vi "AutoMessageFGV.vi"(6 "Timeout (ms)":i32=-1, 8 "error in (no error)":errorcluster, 11 "VI Refnum In":refnum<vi>) -> (0 "error out":errorcluster, 3 "VI Refnum Out":refnum<vi>)   [LabVIEW 2019, in "MicronTemplateAPIs.lvlib" / "MicronTemplateAPIs.lvclass"]
uses:
  MicronTemplateAPIs.lvclass
  <vilib>/LabJSON/LabJSON.lvlib
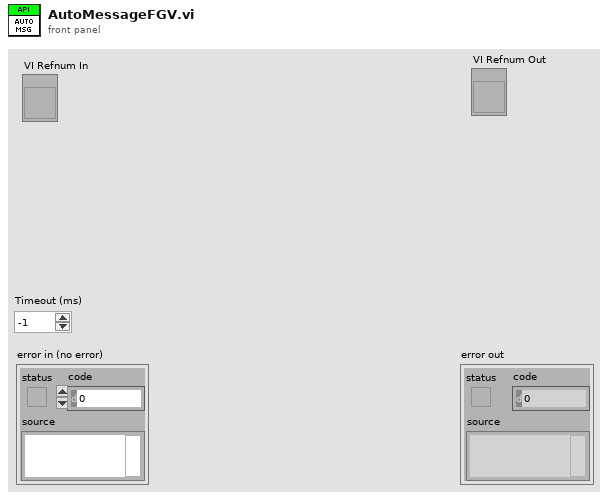
[diagram p1: front panel]
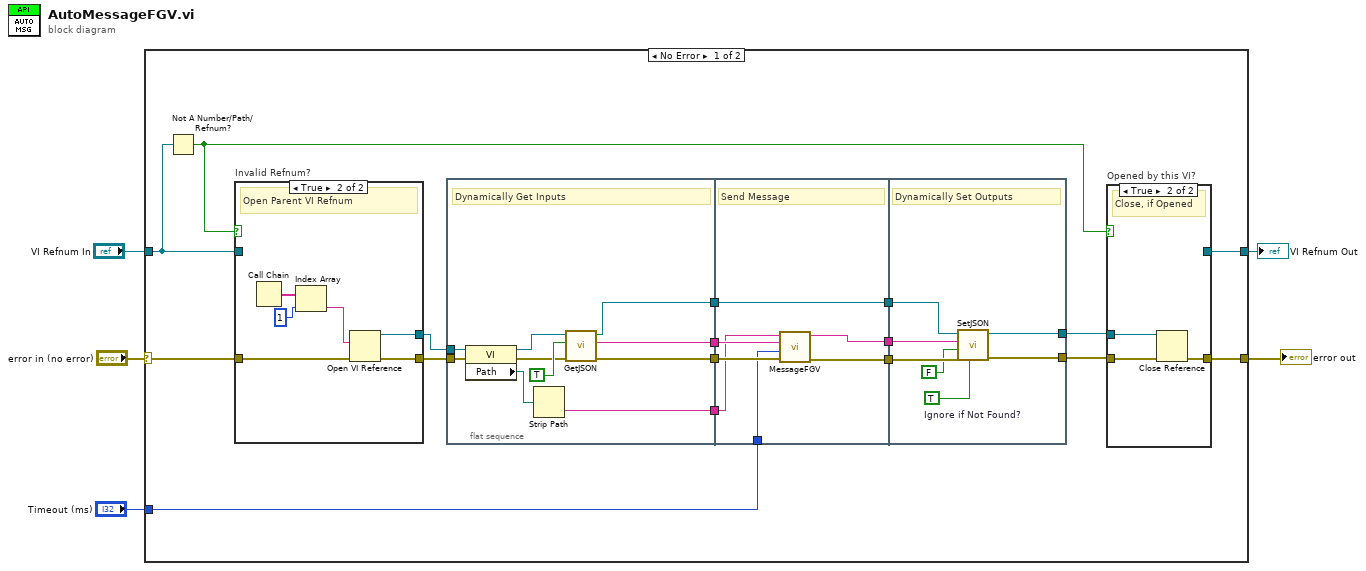
[diagram p0: block diagram]
diagram:
  n1 = case shown="No Error" "error in (no error)" {
    selector: "error in (no error)" -> [w22 w61]
    tunnel: [w19 w61] -> w4
    tunnel: "Timeout (ms)" -> [w11 _]
    tunnel: "VI Refnum In" -> [w20 w60]
    tunnel: [w17 w60] -> w1
    frame No Error {
      n2 = Not A Number/Path/Refnum?(number/path/refnum=w20) -> (NaN/Path/Refnum?=w18:bool)
      n3 = case "Invalid Refnum?" shown="True" w18 {
        tunnel: w22 -> [w52 w57]
        tunnel: [w52 w56] -> w21
        tunnel: [w53 w54] -> w16
        tunnel: w20 -> [w53 _]
        frame False {
        }
        frame True {
          # "Open Parent VI Refnum"
          n4 = Call Chain() -> (call chain=w59:string[])
          n5 = Index Array(array=w59, index=1) -> (element=w55:string)
          n6 = Open VI Reference(vi path=w55, error in (no error)=w57) -> (vi reference=w54:refnum<vi>, error out=w56:errorcluster)  [unwired: 4 in]
        }
      }
      n7 = flat-sequence {
        tunnel: w21 -> [w28]
        tunnel: w16 -> [w26]
        tunnel: [w32] -> w15
        tunnel: [w31] -> w14
        tunnel: [w30] -> w13
        tunnel: [w23] -> w12
        tunnel: w15 -> [w38]
        tunnel: w14 -> [w39]
        tunnel: w13 -> [w36]
        tunnel: w12 -> [w35]
        tunnel: w11 -> [w37]
        tunnel: [w39] -> w10
        tunnel: [w34] -> w9
        tunnel: [w33] -> w8
        tunnel: w10 -> [w43]
        tunnel: w9 -> [w46]
        tunnel: w8 -> [w44]
        tunnel: [w42] -> w7
        tunnel: [w41] -> w6
        frame #0 {
          # "Dynamically Get Inputs"
          n8 = property class="VI"(reference=w26, error in=w28) -> (reference out=w25:refnum<vi>, error out=w27:errorcluster, "Path"=w24:path)
          n9 = Strip Path(path=w24) -> (name=w23:string)  [unwired: 1 out]
          n10 = call <vilib>:"GetJSON.vi"("Error In"=w27, "Controls?"=TRUE, "VI Refnum In"=w25) -> ("Error Out"=w32:errorcluster, "JSON Out"=w30:string, "VI Refnum Out"=w31:refnum<vi>)  [unwired: 6 in]
        }
        frame #1 {
          # "Send Message"
          n11 = call "MessageFGV.vi"("error in (no error)"=w38, "Timeout (ms)"=w37, "Payload"=w36, "Command"=w35) -> ("error out"=w34:errorcluster, "Response"=w33:string)  [unwired: 6 in]
        }
        frame #2 {
          w40 = TRUE  # Ignore if Not Found?
          # "Dynamically Set Outputs"
          n12 = call <vilib>:"SetJSON.vi"("Ignore if Not Found?"=w40, "Error In"=w46, "Controls?"=FALSE, "JSON Input"=w44, "VI Refnum In"=w43) -> ("Error Out"=w42:errorcluster, "VI Refnum Out"=w41:refnum<vi>)  [unwired: 5 in]
        }
      }
      n13 = case "Opened by this VI?" shown="True" w18 {
        tunnel: w7 -> [w48 w51]
        tunnel: [w48 w50] -> w19
        tunnel: w6 -> [w47 w49]
        tunnel: [w47 _] -> w17
        frame False {
        }
        frame True {
          # "Close, if Opened"
          n14 = Close Reference(reference=w49, error in (no error)=w51) -> (error out=w50:errorcluster)
        }
      }
    }
    frame Error {
    }
  }
  "error out" <- w4
  "VI Refnum Out" <- w1
